vi "Power Output Update Ranges Listbox.vi"(6 "Colors":cluster{"Pass":u32, "Fail":u32, "Nop":u32}={"Pass"=6618880, "Fail"=16711680, "Nop"=16777226}, 7 "State (Pass/Fail)":enum16{"Reset", "In Progress", "Pass/Fail"}(ring), 8 "error in (no error)":errorcluster, 9 "Pass/Fail":bool[](array[boolean]), 10 "Stimulus":T1, 11 "Ranges Measured":refnum<vi>) -> (0 "error out":errorcluster, 3 "Ranges Measured":refnum<vi>)   [LabVIEW 2011]
uses:
  TypeDefs/Power Output Stimulus Parameters.ctl
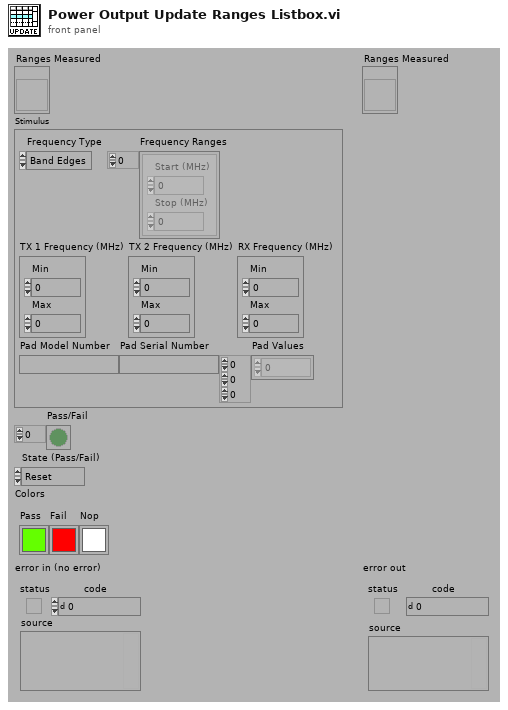
[diagram p1: front panel]
types:
  T1 = typedef "Power Output Stimulus Parameters.ctl" = cluster{"Frequency Type":enum16{"Band Edges", "Custom"}, "Frequency Ranges":cluster{"Start (MHz)":dbl, "Stop (MHz)":dbl}[], "TX 1 Frequency (MHz)":cluster{"Min":dbl, "Max":dbl}, "TX 2 Frequency (MHz)":cluster{"Min":dbl, "Max":dbl}, "RX Frequency (MHz)":cluster{"Min":dbl, "Max":dbl}, "Pad Model Number":string, "Pad Serial Number":string, "Pad Values":dbl[][][]}
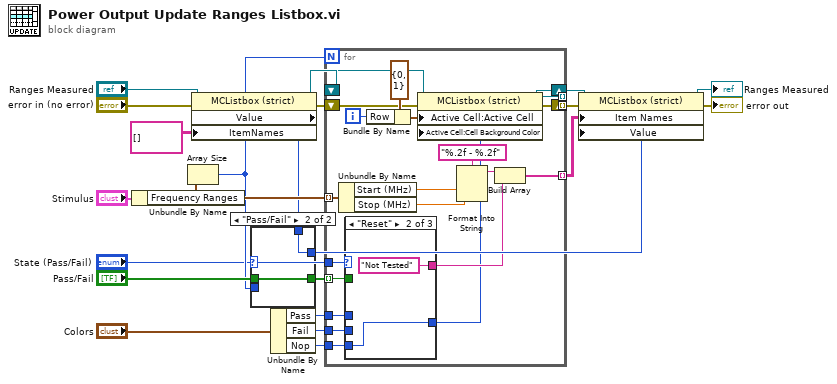
[diagram p0: block diagram]
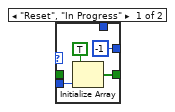
[diagram p2: hidden frame]
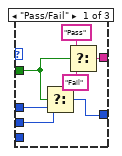
[diagram p3: hidden frame]
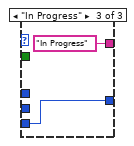
[diagram p4: hidden frame]
diagram:
  n1 = Unbundle By Name("Stimulus") -> ("Frequency Ranges"=w15:cluster{"Start (MHz)":dbl, "Stop (MHz)":dbl}[])
  n2 = Array Size(array=w15) -> (size(s)=w14:i32)
  n3 = property class="MCListbox (strict)"(reference="Ranges Measured", error in="error in (no error)", "ItemNames"=string[][] [] ("Item Names")) -> (reference out=w10:refnum<vi>, error out=w9:errorcluster, "Value"=w1:i32)
  n4 = case shown="\"Pass/Fail\"" "State (Pass/Fail)" {
    tunnel: [w25 w28] -> w18
    tunnel: "Pass/Fail" -> [_ w28]
    tunnel: w14 -> [w24 _]
    tunnel: [-1 ("Value") w27] -> w2
    tunnel: w1 -> [_ w27]
    frame "Reset", "In Progress" {
      n5 = Initialize Array(TRUE, w24) -> (w25:bool[])
    }
    frame "Pass/Fail" {
    }
  }
  n6 = Unbundle By Name("Colors") -> ("Pass"=w21:u32, "Fail"=w20:u32, "Nop"=w19:u32)
  n7 = for {
    N: w14 -> [_]
    tunnel: w21 -> [w39]
    tunnel: w20 -> [w38]
    shift-right: [w32] -> w7
    shift-left: w9 -> [w45]
    tunnel: [w44] -> w5 mode=indexing
    tunnel: w18 -> [w37] mode=indexing
    tunnel: w19 -> [w35]
    tunnel: "State (Pass/Fail)" -> [w36]
    tunnel: w15 -> [w31] mode=indexing
    shift-right: [w33] -> w6
    shift-left: w10 -> [w46]
    tunnel: [w33] -> _ mode=indexing
    tunnel: [w32] -> _ mode=indexing
    i -> [w34]
    n8 = Unbundle By Name(w31) -> ("Start (MHz)"=w30:dbl, "Stop (MHz)"=w29:dbl)
    n9 = case shown="\"Reset\"" w36 {
      tunnel: [w51 "Not Tested" "In Progress"] -> w41
      tunnel: [w55 w56 w58] -> w40
      tunnel: w39 -> [w54 _ _]
      tunnel: w38 -> [w53 _ _]
      tunnel: w37 -> [w52 _ _]
      tunnel: w35 -> [_ w56 w58]
      frame "Pass/Fail" {
        n10 = Select(t=w54, s=w52, f=w53) -> (s? t:f=w55:u32)
        n11 = Select(t="Pass" ("format string"), s=w52, f="Fail" ("format string")) -> (s? t:f=w51:string)
      }
      frame "Reset" {
      }
      frame "In Progress" {
      }
    }
    n12 = Bundle By Name(cluster=cluster{"Row":i32, "Column":i32} {"Row"=0, "Column"=1} ("Active Cell"), "Row"=w34) -> (w47:cluster{"Row":i32, "Column":i32})
    n13 = property class="MCListbox (strict)"(reference=w46, error in=w45, "Active Cell:Active Cell"=w47, "Active Cell:Cell Background Color"=w40) -> (reference out=w33:refnum<vi>, error out=w32:errorcluster)
    n14 = Format Into String(format string="%.2f - %.2f", w30, w29) -> (resulting string=w42:string)  [unwired: 2 in, 1 out]
    n15 = Build Array(w42, w41) -> (w44:string[])
  }
  n16 = property class="MCListbox (strict)"(reference=w6, error in=w7, "Item Names"=w5, "Value"=w2) -> (reference out=→"Ranges Measured":refnum<vi>, error out=→"error out":errorcluster)
